vi "Callback - Set Value.vi"(10 "Value":dbl, 11 "Number Widget in":refnum<class "LQObject.lvclass">) -> ()   [LabVIEW 2013, in "6. Number Widget.lvclass"]
doc: "Copyright (c) 2016 Sze Howe Koh\nThis code is licensed under the MIT license"
uses:
  6. Number Widget.lvclass
  src/LabVIEW/LQ Core/LQObject/LQObject.lvclass
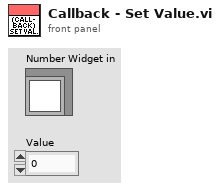
[diagram p1: front panel]
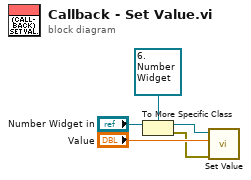
[diagram p0: block diagram]
diagram:
  n1 = To More Specific Class(target class=refnum<class "6. Number Widget.lvclass"> refnum ("Number Widget"), reference="Number Widget in") -> (specific class reference=w3:refnum<class "6. Number Widget.lvclass">, error out=w1:errorcluster)  [unwired: 1 in]
  n2 = call "Set Value.vi"("Error In"=w1, "Value"="Value", "Number Widget In"=w3) -> ()  [unwired: 7 in, 2 out]
